vi "Write Identifier.vi"(8 "error in (no error)":errorcluster, 10 "identifier":u32, 11 "Session Handle in":T1) -> (0 "error out":errorcluster, 3 "Session Handle out":T1)   [LabVIEW 2015, in "Oil.lvclass"]
uses:
  Oil.lvclass
  Typedefs/Session Handle.ctl
  Oil.lvclass/Oil.ctl
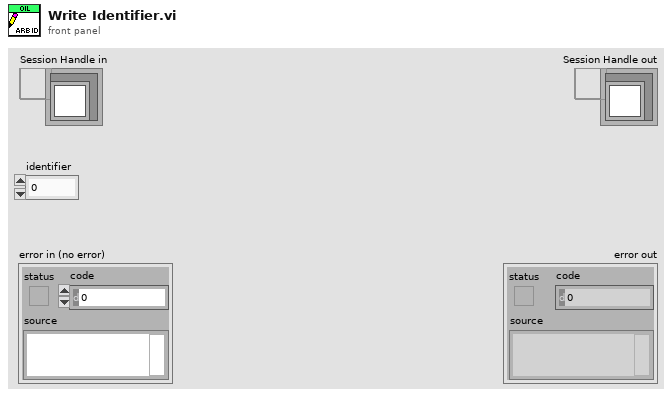
[diagram p1: front panel]
types:
  T1 = typedef "Oil.lvclass/Session Handle.ctl" = refnum<data-value>
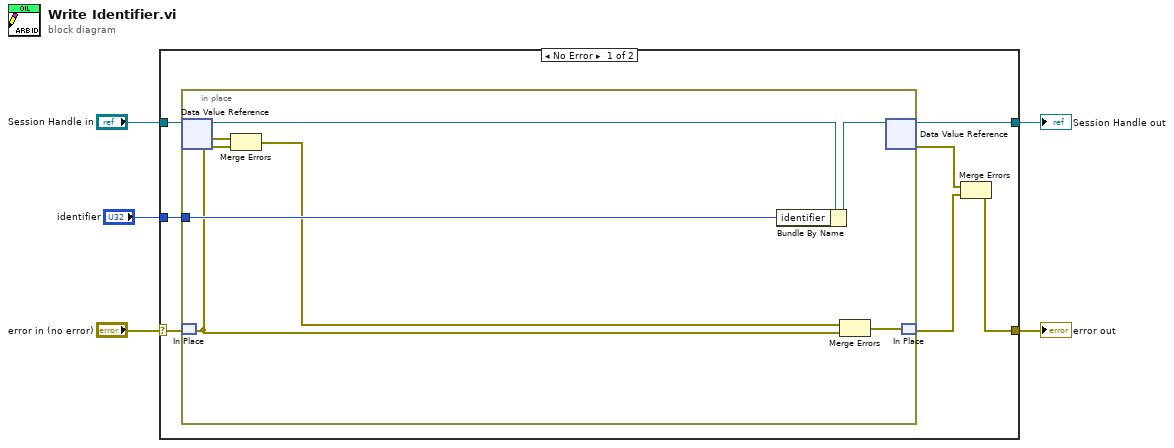
[diagram p0: block diagram]
diagram:
  n1 = case shown="No Error" "error in (no error)" {
    selector: "error in (no error)" -> [w7 w20]
    tunnel: "Session Handle in" -> [w12 w21]
    tunnel: [w11 w21] -> w4
    tunnel: [w8 w20] -> w3
    tunnel: "identifier" -> [w6 _]
    frame No Error {
      n2 = in-place {
        in-place-border: w6 -> [w15]
        n3 = in-place-dvr #1(w12) -> (w18:refnum<class "Oil.lvclass">, w19:errorcluster)
        n4 = in-place-match #2(w7) -> (w14:errorcluster)
        n5 = Merge Errors(w14, w19) -> (w13:errorcluster)
        n6 = Bundle By Name(cluster=w18, "identifier"=w15) -> (w17:refnum<class "Oil.lvclass">)
        n7 = Merge Errors(w13, w14) -> (w16:errorcluster)
        n8 = in-place-dvr #1(w17) -> (w11:T1, w9:errorcluster)
        n9 = in-place-match #2(w16) -> (w10:errorcluster)
      }
      n10 = Merge Errors(w9, w10) -> (w8:errorcluster)
    }
    frame Error {
    }
  }
  "Session Handle out" <- w4
  "error out" <- w3
